vi "Motor Not Running--error.vi"() -> (0 "error out":errorcluster)   [LabVIEW 2024, in "Clon.lvlib"]
uses:
  Clon.lvlib
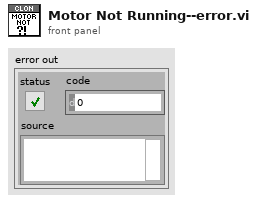
[diagram p1: front panel]
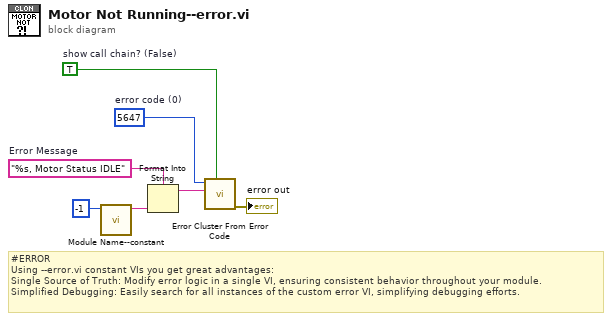
[diagram p0: block diagram]
diagram:
  w5 = 5647  # error code (0)
  w3 = "%s, Motor Status IDLE"  # Error Message
  w6 = TRUE  # show call chain? (False)
  # "#ERROR\nUsing --error.vi constant VIs you get great advantages:\nSingle Source of Truth: Modify error logic in a single VI, ensuring consistent behavior throughout your module.\nSimplified Debugging: Easily search for all instances of the custom error VI, simplifying debugging efforts."
  n1 = call "Module Name--constant.vi"("Module ID"=-1) -> ("Module Name"=w2:string)  [unwired: 10 in]
  n2 = Format Into String(format string=w3, w2) -> (resulting string=w4:string)  [unwired: 2 in, 1 out]
  n3 = call <vilib>:"Error Cluster From Error Code.vi"("show call chain? (False)"=w6, "error message (\"\")"=w4, "error code (0)"=w5) -> ("error out"=→"error out":errorcluster)  [unwired: 6 in]
